vi "Test_UpdateChannelsList.vi"() -> ()   [LabVIEW 2019]
uses:
  ByteQXAPIBase/ByteQXAPIBase.lvclass
panel:
  out "test passed?":bool
  out "error out":errorcluster
  in  "channels":string[](array[string])
  in  "asset code":string
  in  "Auth token":string
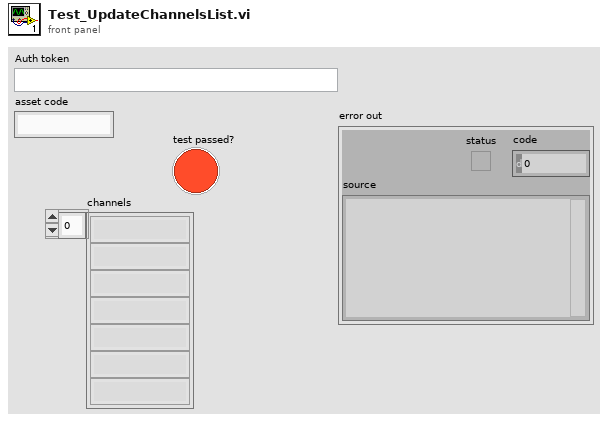
[diagram p1: front panel]
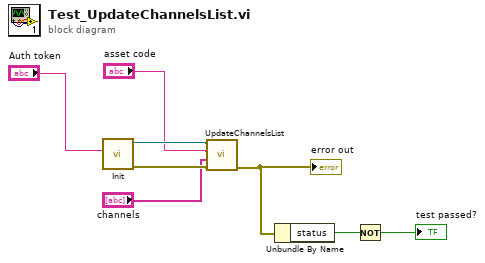
[diagram p0: block diagram]
diagram:
  n1 = call "Init.vi"("Auth token"="Auth token") -> ("error out"=w4:errorcluster, "ByteQXAPIBase out"=w5:refnum<class "ByteQXAPIBase.lvclass">)  [unwired: 9 in]
  n2 = call "UpdateChannelsList.vi"("error in (no error)"=w4, "channels"="channels", "asset code"="asset code", "ByteQXAPIBase in"=w5) -> ("error out"=w1:errorcluster)  [unwired: 6 in, 1 out]
  "error out" <- w1
  n3 = Unbundle By Name(w1) -> ("status"=w7:bool)
  n4 = Not(x=w7) -> (.not. x?=→"test passed?":bool)
